vi "EEC EST 300 Creating and Saving a File.vi"(0 "VISA resource name":refnum<visa-resource-name>="COM1", 1 "Internal scanner?":bool, 5 "File Name":string="RandomT", 11 "error in (no error)":errorcluster) -> (4 "Error Occured?":bool, 15 "error out":errorcluster)   [LabVIEW 2020]
doc: "This VI is an example on how to Create and Save files in the EPV 500 series.\n\nIt will create a file called \"RandomT\" and fill it with default DCW, IR,GND,PID test types."
uses:
  <instrlib>/eec EST 300/Public/Configure/Steps/Low Level/DCW Test Parameters.ctl
  <instrlib>/eec EST 300/Public/Configure/Steps/Low Level/Scanner Settings.ctl
  <instrlib>/eec EST 300/Public/Configure/Steps/Low Level/IR Test Parameters.ctl
  <instrlib>/eec EST 300/eec EST 300.lvlib
panel:
  in  "Scanner Settings":T1={"Scan1"=1, "Scan2"=1, "Scan3"=1, "Scan4"=1, "Scan5"=1, "Scan6"=1, "Scan7"=1, "Scan8"=1, "Scan9"=1, "Scan10"=1, "Scan11"=1, "Scan12"=1, "Scan13"=1, "Scan14"=1, "Scan15"=1, "Scan16"=1} {"Scan16" scale=0.0..2.0; "Scan15" scale=0.0..2.0; "Scan14" scale=0.0..2.0; "Scan13" scale=0.0..2.0; "Scan12" scale=0.0..2.0; "Scan11" scale=0.0..2.0; "Scan10" scale=0.0..2.0; "Scan9" scale=0.0..2.0; "Scan8" scale=0.0..2.0; "Scan7" scale=0.0..2.0; "Scan6" scale=0.0..2.0; "Scan5" scale=0.0..2.0; "Scan4" scale=0.0..2.0; "Scan3" min=0 max=2 scale=0.0..2.0; "Scan2" min=0 max=2 scale=0.0..2.0; "Scan1" min=0 max=2 scale=0.0..2.0}
  in  "IR Test Parameters":T2={"Voltage (10~3000V)"=500, "High Limit(0.0, 0.1~50,000 Mohms)"=0.0, "Low Limit(0.1~50,000 Mohms)"=10.0, "Ramp Up Time (0.1~999.9 seconds)"=0.1, "Delay Time (0.5~999.9 seconds)"=0.5, "Ramp Down Time (0.0, 1.0~999.9 seconds)"=0.0, "Charge LO  (0.000~3.500uA)"=0.0, "Auto Charge LO (F: Off)"=FALSE, "Dwell Time (0.5~999.9 seconds, 0 = Constant)"=0.5} {"Dwell Time (0.5~999.9 seconds, 0 = Constant)" format="%.1f"; "Ramp Down Time (0.0, 1.0~999.9 seconds)" format="%.1f"; "Charge LO  (0.000~3.500uA)" format="%.3f"; "Delay Time (0.5~999.9 seconds)" format="%.1f"; "Ramp Up Time (0.1~999.9 seconds)" format="%.1f"; "Low Limit(0.1~50,000 Mohms)" format="%.1f"; "High Limit(0.0, 0.1~50,000 Mohms)" format="%.1f"}
  in  "Scanner Settings":T1={"Scan1"=1, "Scan2"=1, "Scan3"=1, "Scan4"=1, "Scan5"=1, "Scan6"=1, "Scan7"=1, "Scan8"=1, "Scan9"=1, "Scan10"=1, "Scan11"=1, "Scan12"=1, "Scan13"=1, "Scan14"=1, "Scan15"=1, "Scan16"=1} {"Scan16" scale=0.0..2.0; "Scan15" scale=0.0..2.0; "Scan14" scale=0.0..2.0; "Scan13" scale=0.0..2.0; "Scan12" scale=0.0..2.0; "Scan11" scale=0.0..2.0; "Scan10" scale=0.0..2.0; "Scan9" scale=0.0..2.0; "Scan8" scale=0.0..2.0; "Scan7" scale=0.0..2.0; "Scan6" scale=0.0..2.0; "Scan5" scale=0.0..2.0; "Scan4" scale=0.0..2.0; "Scan3" min=0 max=2 scale=0.0..2.0; "Scan2" min=0 max=2 scale=0.0..2.0; "Scan1" min=0 max=2 scale=0.0..2.0}
  in  "DCW Test Parameters":T3={"Voltage (0~6.0 KV)"=1.0, "High Limit(0.0~7500 uA)"=10.0, "Low Limit(0~7500 uA)"=0.0, "Ramp Up Time (0.1~999.9 seconds)"=0.4, "Dwell Time (0, 0.4~999.9 seconds)"=1.0, "Ramp Down Time (0, 1.0~999.9 seconds)"=0.0, "Charge LO (0.0~350uA)"=0.0, "Arc Sense (1~9)"=5, "Arc Detect (F: Off)"=FALSE, "Auto Charge LO (F: Off)"=FALSE, "Ramp-Hi (0.0~7500 uA)"=0.0} {"Ramp-Hi (0.0~7500 uA)" format="%.2f"; "Ramp Down Time (0, 1.0~999.9 seconds)" format="%.1f"; "Charge LO (0.0~350uA)" format="%.2f"; "Dwell Time (0, 0.4~999.9 seconds)" format="%.1f"; "Ramp Up Time (0.1~999.9 seconds)" format="%.1f"; "Low Limit(0~7500 uA)" format="%.1f"; "High Limit(0.0~7500 uA)" format="%.1f"; "Voltage (0~6.0 KV)" format="%.2f"}
  # "On\nOff"
  # "On\nOff"
  # "On\nOff"
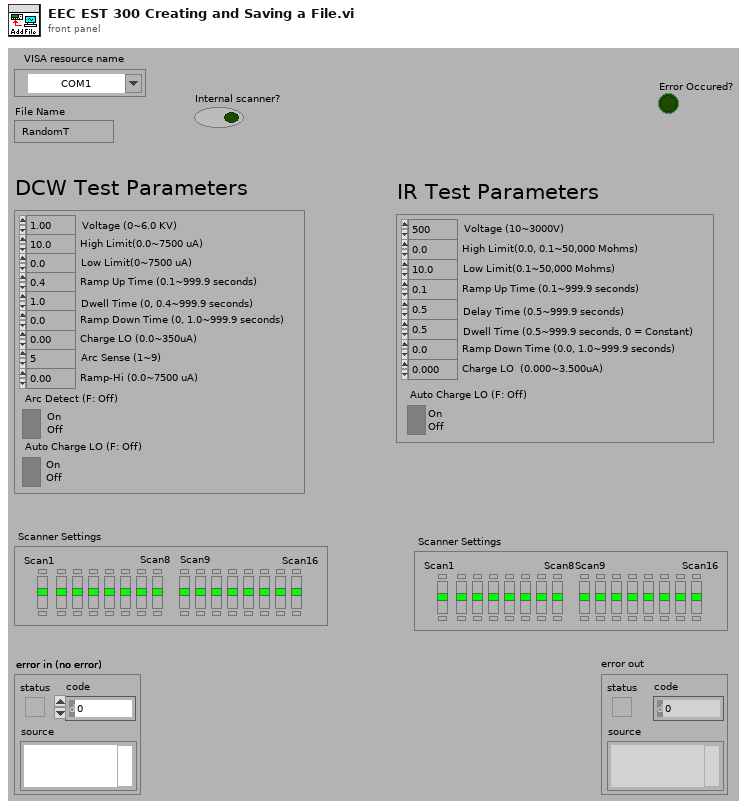
[diagram p1: front panel]
types:
  T1 = typedef "EEC EST 300.lvlib/Scanner Settings.ctl" = cluster{"Scan1":i32, "Scan2":i32, "Scan3":i32, "Scan4":i32, "Scan5":i32, "Scan6":i32, "Scan7":i32, "Scan8":i32, "Scan9":i32, "Scan10":i32, "Scan11":i32, "Scan12":i32, "Scan13":i32, "Scan14":i32, "Scan15":i32, "Scan16":i32}
  T2 = typedef "EEC EST 300.lvlib/IR Test Parameters.ctl" = cluster{"Voltage (10~3000V)":i64, "High Limit(0.0, 0.1~50,000 Mohms)":dbl, "Low Limit(0.1~50,000 Mohms)":dbl, "Ramp Up Time (0.1~999.9 seconds)":dbl, "Delay Time (0.5~999.9 seconds)":dbl, "Ramp Down Time (0.0, 1.0~999.9 seconds)":dbl, "Charge LO  (0.000~3.500uA)":dbl, "Auto Charge LO (F: Off)":bool, "Dwell Time (0.5~999.9 seconds, 0 = Constant)":dbl}
  T3 = typedef "eec EST 300.lvlib/DCW Test Parameters.ctl" = cluster{"Voltage (0~6.0 KV)":dbl, "High Limit(0.0~7500 uA)":dbl, "Low Limit(0~7500 uA)":dbl, "Ramp Up Time (0.1~999.9 seconds)":dbl, "Dwell Time (0, 0.4~999.9 seconds)":dbl, "Ramp Down Time (0, 1.0~999.9 seconds)":dbl, "Charge LO (0.0~350uA)":dbl, "Arc Sense (1~9)":i32, "Arc Detect (F: Off)":bool, "Auto Charge LO (F: Off)":bool, "Ramp-Hi (0.0~7500 uA)":dbl}
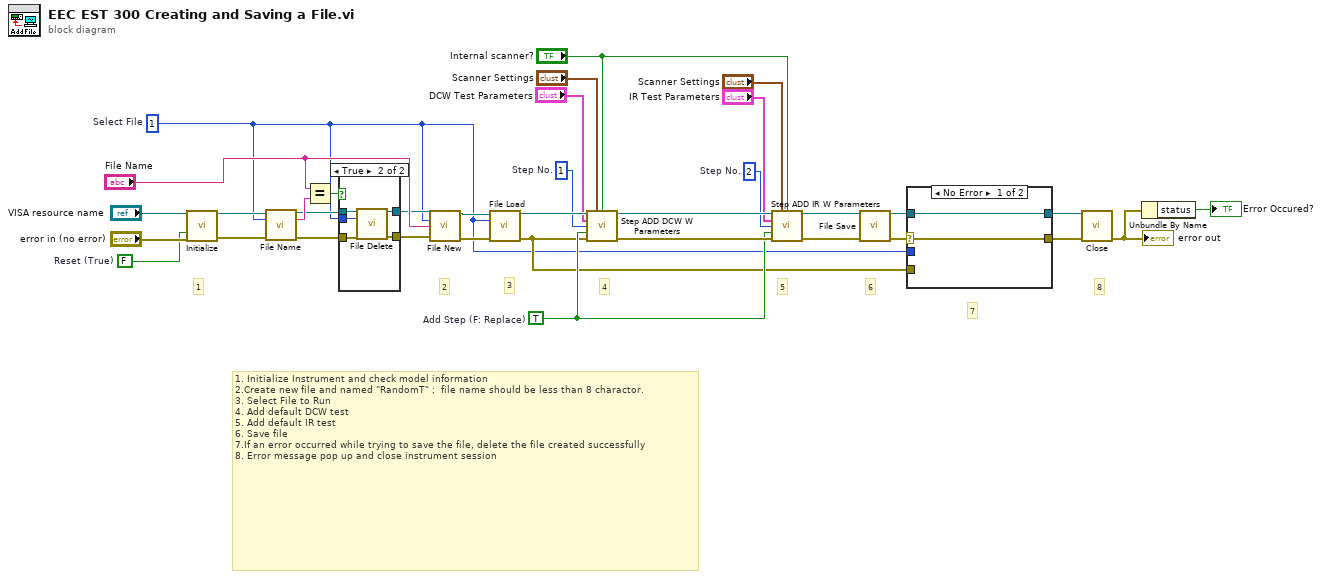
[diagram p0: block diagram]
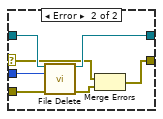
[diagram p3: hidden frame]
diagram:
  w21 = 2  # Step No.
  w28 = 1  # Step No.
  w22 = TRUE  # Add Step (F: Replace)
  w1 = 1  # Select File
  w33 = FALSE  # Reset (True)
  # "7"
  # "8"
  # "6"
  # "5"
  # "4"
  # "1. Initialize Instrument and check model information\n2.Create new file and named \"RandomT\" ;  file name should be less than 8 charactor.\n3. Select File to Run\n4. Add default DCW test\n5. Add default IR test\n6. Save file\n7.If an error occurred while trying to save the file, delete the file created successfully\n8. Error message pop up and close instrument session"
  # "3"
  # "2"
  # "1"
  n1 = call <instrlib>:"Initialize.vi"("VISA resource name"="VISA resource name", "Reset (True)"=w33, "error in (no error)"="error in (no error)") -> ("VISA resource name out"=w10:refnum<visa-resource-name>, "error out"=w9:errorcluster)  [unwired: 10 in, 1 out]
  n2 = call <instrlib>:"File Name.vi"("VISA resource name"=w10, "File Number"=w1, "error in (no error)"=w9) -> ("VISA resource name out"=w5:refnum<visa-resource-name>, "File Name"=w8:string, "error out"=w4:errorcluster)  [unwired: 10 in]
  n3 = Equal?(x="File Name", y=w8) -> (x = y?=w6:bool)
  n4 = case shown="True" w6 {
    tunnel: w5 -> [w37 w41]
    tunnel: w4 -> [w36 w42]
    tunnel: [w37 w40] -> w3
    tunnel: [w36 w39] -> w2
    tunnel: w1 -> [_ w38]
    frame False {
    }
    frame True {
      n5 = call <instrlib>:"File Delete.vi"("VISA resource name"=w41, "File Number"=w38, "error in (no error)"=w42) -> ("VISA resource name out"=w40:refnum<visa-resource-name>, "error out"=w39:errorcluster)  [unwired: 11 in]
    }
  }
  n6 = call <instrlib>:"File New.vi"("VISA resource name"=w3, "File Number"=w1, "File Name"="File Name", "error in (no error)"=w2) -> ("VISA resource name out"=w30:refnum<visa-resource-name>, "error out"=w27:errorcluster)  [unwired: 10 in]
  n7 = call <instrlib>:"File Load.vi"("VISA resource name"=w30, "File Number (1-2000)"=w1, "error in (no error)"=w27) -> ("VISA resource name out"=w29:refnum<visa-resource-name>, "error out"=w15:errorcluster)  [unwired: 11 in]
  n8 = call <instrlib>:"Step ADD DCW W Parameters.vi"("VISA resource name"=w29, "Scanner Settings"="Scanner Settings", "Internal scanner?"="Internal scanner?", "DCW Test Parameters (in)"="DCW Test Parameters", "Step Selection (1-200)"=w28, "Add Step"=w22, "error in (no error)"=w15) -> ("VISA resource name out"=w24:refnum<visa-resource-name>, "error out"=w23:errorcluster)  [unwired: 7 in]
  n9 = call <instrlib>:"Step ADD IR W Parameters.vi"("VISA resource name"=w24, "Scanner Settings"="Scanner Settings", "Internal scanner?"="Internal scanner?", "IR Test Parameters In"="IR Test Parameters", "Step Selection (1-200)"=w21, "Add Step"=w22, "error in (no error)"=w23) -> ("VISA resource name out"=w12:refnum<visa-resource-name>, "error out"=w11:errorcluster)  [unwired: 7 in]
  n10 = call <instrlib>:"File Save.vi"("VISA resource name"=w12, "error in (no error)"=w11) -> ("VISA resource name out"=w16:refnum<visa-resource-name>, "error out"=w17:errorcluster)  [unwired: 12 in]
  n11 = case shown="No Error" w17 {
    selector: w17 -> [w44 w46]
    tunnel: w16 -> [w43 w50]
    tunnel: w15 -> [_ w51]
    tunnel: [w44 w45] -> w14
    tunnel: [w43 w49] -> w13
    tunnel: w1 -> [_ w48]
    frame No Error {
    }
    frame Error {
      n12 = call <instrlib>:"File Delete.vi"("VISA resource name"=w50, "File Number"=w48, "error in (no error)"=w51) -> ("VISA resource name out"=w49:refnum<visa-resource-name>, "error out"=w47:errorcluster)  [unwired: 11 in]
      n13 = Merge Errors(w46, w47) -> (w45:errorcluster)
    }
  }
  n14 = call <instrlib>:"Close.vi"("VISA resource name"=w13, "error in (no error)"=w14) -> ("error out"=w31:errorcluster)  [unwired: 13 in]
  "error out" <- w31
  n15 = Unbundle By Name(w31) -> ("status"=→"Error Occured?":bool)
